vi "(SubVI) Write to Three Axises_YCC.vi"(2 "handle":i32, 4 "Position wrote to three axis (um)":dbl) -> ()   [LabVIEW 2014]
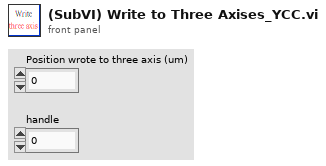
[diagram p1: front panel]
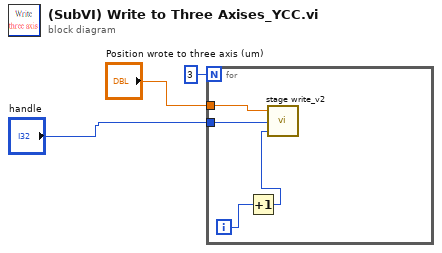
[diagram p0: block diagram]
diagram:
  n1 = for {
    N: 3 -> [_]
    tunnel: "handle" -> [w5]
    tunnel: "Position wrote to three axis (um)" -> [w4]
    i -> [w7]
    n2 = Increment(x=w7) -> (x+1=w6:i32)
    n3 = call "stage write_v2.vi"("axis"=w6, "Incoming Handle"=w5, "position"=w4) -> ()  [unwired: 2 in, 1 out]
  }
